vi "Sonatina.vi"(11 "NXT/EV3":T1) -> (3 "NXT/EV3 2":T1)   [LabVIEW 2016]
uses:
  <vilib>/NXT/Subs/LVHSConnector.ctl
  <vilib>/NXT/LegoClasses/BrickReference/BrickReference.lvclass
  <vilib>/NXT/Dual Mode Library/Display/drawText_Center.vi
  <vilib>/NXT/Dual Mode Library/Sound/PlayG.vi
  <vilib>/NXT/Dual Mode Library/Waits/Wait_Num.vi
  <vilib>/NXT/Dual Mode Library/Sound/PlayB.vi
  <vilib>/NXT/Dual Mode Library/Sound/PlayA.vi
  <vilib>/NXT/Dual Mode Library/Sound/PlayD.vi
  <vilib>/NXT/Dual Mode Library/Sound/PlayC.vi
  <vilib>/NXT/Dual Mode Library/Sound/PlayE.vi
  <vilib>/NXT/Dual Mode Library/Sound/PlayFsharp.vi
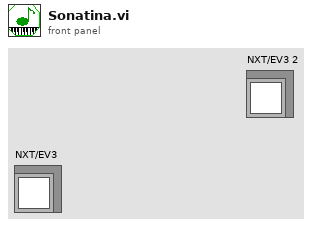
[diagram p1: front panel]
types:
  T1 = typedef "LVHSConnector.ctl" = refnum<class "BrickReference.lvclass">
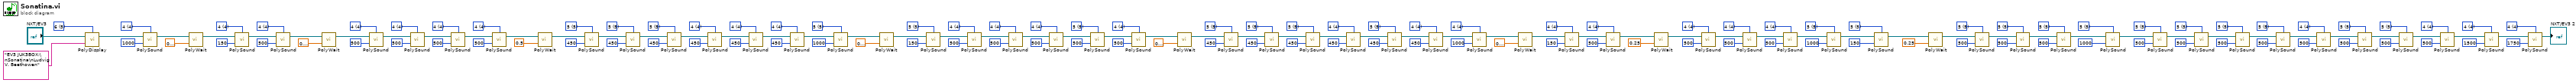
[diagram p0: block diagram]
diagram:
  w5 = u16 4 items=["3"=3, "4"=4, "5"=5, "6"=6, "7"=7] ("Octave")
  w9 = u16 5 items=["3"=3, "4"=4, "5"=5, "6"=6, "7"=7] ("Octave")
  w16 = u16 4 items=["3"=3, "4"=4, "5"=5, "6"=6, "7"=7] ("Octave")
  w19 = u16 4 items=["3"=3, "4"=4, "5"=5, "6"=6, "7"=7] ("Octave")
  w20 = u16 5 items=["3"=3, "4"=4, "5"=5, "6"=6, "7"=7] ("Octave")
  w23 = u16 4 items=["3"=3, "4"=4, "5"=5, "6"=6, "7"=7] ("Octave")
  w24 = u16 5 items=["3"=3, "4"=4, "5"=5, "6"=6, "7"=7] ("Octave")
  w27 = u16 5 items=["3"=3, "4"=4, "5"=5, "6"=6, "7"=7] ("Octave")
  w28 = u16 5 items=["3"=3, "4"=4, "5"=5, "6"=6, "7"=7] ("Octave")
  w31 = u16 5 items=["3"=3, "4"=4, "5"=5, "6"=6, "7"=7] ("Octave")
  w41 = u16 5 items=["3"=3, "4"=4, "5"=5, "6"=6, "7"=7] ("Octave")
  w40 = u16 5 items=["3"=3, "4"=4, "5"=5, "6"=6, "7"=7] ("Octave")
  w37 = u16 5 items=["3"=3, "4"=4, "5"=5, "6"=6, "7"=7] ("Octave")
  w36 = u16 5 items=["3"=3, "4"=4, "5"=5, "6"=6, "7"=7] ("Octave")
  w33 = u16 5 items=["3"=3, "4"=4, "5"=5, "6"=6, "7"=7] ("Octave")
  w61 = u16 5 items=["3"=3, "4"=4, "5"=5, "6"=6, "7"=7] ("Octave")
  w62 = u16 4 items=["3"=3, "4"=4, "5"=5, "6"=6, "7"=7] ("Octave")
  w65 = u16 4 items=["3"=3, "4"=4, "5"=5, "6"=6, "7"=7] ("Octave")
  w66 = u16 4 items=["3"=3, "4"=4, "5"=5, "6"=6, "7"=7] ("Octave")
  w69 = u16 4 items=["3"=3, "4"=4, "5"=5, "6"=6, "7"=7] ("Octave")
  w70 = u16 4 items=["3"=3, "4"=4, "5"=5, "6"=6, "7"=7] ("Octave")
  w73 = u16 4 items=["3"=3, "4"=4, "5"=5, "6"=6, "7"=7] ("Octave")
  w83 = u16 4 items=["3"=3, "4"=4, "5"=5, "6"=6, "7"=7] ("Octave")
  w84 = u16 5 items=["3"=3, "4"=4, "5"=5, "6"=6, "7"=7] ("Octave")
  w86 = u16 4 items=["3"=3, "4"=4, "5"=5, "6"=6, "7"=7] ("Octave")
  w89 = u16 5 items=["3"=3, "4"=4, "5"=5, "6"=6, "7"=7] ("Octave")
  w90 = u16 5 items=["3"=3, "4"=4, "5"=5, "6"=6, "7"=7] ("Octave")
  w93 = u16 5 items=["3"=3, "4"=4, "5"=5, "6"=6, "7"=7] ("Octave")
  w95 = u16 4 items=["3"=3, "4"=4, "5"=5, "6"=6, "7"=7] ("Octave")
  w110 = u16 5 items=["3"=3, "4"=4, "5"=5, "6"=6, "7"=7] ("Octave")
  w107 = u16 4 items=["3"=3, "4"=4, "5"=5, "6"=6, "7"=7] ("Octave")
  w106 = u16 4 items=["3"=3, "4"=4, "5"=5, "6"=6, "7"=7] ("Octave")
  w103 = u16 4 items=["3"=3, "4"=4, "5"=5, "6"=6, "7"=7] ("Octave")
  w102 = u16 5 items=["3"=3, "4"=4, "5"=5, "6"=6, "7"=7] ("Octave")
  w99 = u16 5 items=["3"=3, "4"=4, "5"=5, "6"=6, "7"=7] ("Octave")
  w123 = u16 4 items=["3"=3, "4"=4, "5"=5, "6"=6, "7"=7] ("Octave")
  w126 = u16 4 items=["3"=3, "4"=4, "5"=5, "6"=6, "7"=7] ("Octave")
  w130 = u16 4 items=["3"=3, "4"=4, "5"=5, "6"=6, "7"=7] ("Octave")
  w127 = u16 5 items=["3"=3, "4"=4, "5"=5, "6"=6, "7"=7] ("Octave")
  w133 = u16 5 items=["3"=3, "4"=4, "5"=5, "6"=6, "7"=7] ("Octave")
  w136 = u16 5 items=["3"=3, "4"=4, "5"=5, "6"=6, "7"=7] ("Octave")
  w149 = u16 4 items=["3"=3, "4"=4, "5"=5, "6"=6, "7"=7] ("Octave")
  w150 = u16 4 items=["3"=3, "4"=4, "5"=5, "6"=6, "7"=7] ("Octave")
  w153 = u16 4 items=["3"=3, "4"=4, "5"=5, "6"=6, "7"=7] ("Octave")
  w154 = u16 4 items=["3"=3, "4"=4, "5"=5, "6"=6, "7"=7] ("Octave")
  w157 = u16 4 items=["3"=3, "4"=4, "5"=5, "6"=6, "7"=7] ("Octave")
  w158 = u16 4 items=["3"=3, "4"=4, "5"=5, "6"=6, "7"=7] ("Octave")
  w161 = u16 4 items=["3"=3, "4"=4, "5"=5, "6"=6, "7"=7] ("Octave")
  w163 = i16 5 items=["1", "2", "3", "4", "5", "6", "7", "8", "9", "10", "11", "12"] ("Line")
  n1 = call-poly <vilib>:"PolyDisplay.vi"("Text"="EV3 JUK3BOX:\nSonatina\nLudvig V. Beethowen", "NXT/EV3"="NXT/EV3", "Line"=w163) -> ("NXT/EV3"=w143:T1)  [unwired: 1 in]
  n2 = call-poly <vilib>:"PolySound.vi"("Duration (500 ms)"=u16 1000, "NXT/EV3"=w143, "Octave"=w161) -> ("NXT/EV3"=w140:T1)  [unwired: 1 in]
  n3 = call-poly <vilib>:"PolyWait.vi"("Time (1 sec)"=sgl 0.1, "NXT/EV3"=w140) -> ("NXT/EV3"=w141:T1)  [unwired: 2 in]
  n4 = call-poly <vilib>:"PolySound.vi"("Duration (500 ms)"=u16 150, "NXT/EV3"=w141, "Octave"=w158) -> ("NXT/EV3"=w147:T1)  [unwired: 1 in]
  n5 = call-poly <vilib>:"PolySound.vi"("Duration (500 ms)"=u16 500, "NXT/EV3"=w147, "Octave"=w157) -> ("NXT/EV3"=w138:T1)  [unwired: 1 in]
  n6 = call-poly <vilib>:"PolyWait.vi"("Time (1 sec)"=sgl 0.1, "NXT/EV3"=w138) -> ("NXT/EV3"=w137:T1)  [unwired: 2 in]
  n7 = call-poly <vilib>:"PolySound.vi"("Duration (500 ms)"=u16 500, "NXT/EV3"=w137, "Octave"=w154) -> ("NXT/EV3"=w146:T1)  [unwired: 1 in]
  n8 = call-poly <vilib>:"PolySound.vi"("Duration (500 ms)"=u16 500, "NXT/EV3"=w146, "Octave"=w153) -> ("NXT/EV3"=w145:T1)  [unwired: 1 in]
  n9 = call-poly <vilib>:"PolySound.vi"("Duration (500 ms)"=u16 500, "NXT/EV3"=w145, "Octave"=w150) -> ("NXT/EV3"=w144:T1)  [unwired: 1 in]
  n10 = call-poly <vilib>:"PolySound.vi"("Duration (500 ms)"=u16 500, "NXT/EV3"=w144, "Octave"=w149) -> ("NXT/EV3"=w118:T1)  [unwired: 1 in]
  n11 = call-poly <vilib>:"PolyWait.vi"("Time (1 sec)"=sgl 0.5, "NXT/EV3"=w118) -> ("NXT/EV3"=w119:T1)  [unwired: 2 in]
  n12 = call-poly <vilib>:"PolySound.vi"("Duration (500 ms)"=u16 450, "NXT/EV3"=w119, "Octave"=w136) -> ("NXT/EV3"=w132:T1)  [unwired: 1 in]
  n13 = call-poly <vilib>:"PolySound.vi"("Duration (500 ms)"=u16 450, "NXT/EV3"=w132, "Octave"=w133) -> ("NXT/EV3"=w121:T1)  [unwired: 1 in]
  n14 = call-poly <vilib>:"PolySound.vi"("Duration (500 ms)"=u16 450, "NXT/EV3"=w121, "Octave"=w127) -> ("NXT/EV3"=w131:T1)  [unwired: 1 in]
  n15 = call-poly <vilib>:"PolySound.vi"("Duration (500 ms)"=u16 450, "NXT/EV3"=w131, "Octave"=w130) -> ("NXT/EV3"=w120:T1)  [unwired: 1 in]
  n16 = call-poly <vilib>:"PolySound.vi"("Duration (500 ms)"=u16 450, "NXT/EV3"=w120, "Octave"=w126) -> ("NXT/EV3"=w122:T1)  [unwired: 1 in]
  n17 = call-poly <vilib>:"PolySound.vi"("Duration (500 ms)"=u16 450, "NXT/EV3"=w122, "Octave"=w123) -> ("NXT/EV3"=w98:T1)  [unwired: 1 in]
  n18 = call-poly <vilib>:"PolySound.vi"("Duration (500 ms)"=u16 1000, "NXT/EV3"=w98, "Octave"=w99) -> ("NXT/EV3"=w116:T1)  [unwired: 1 in]
  n19 = call-poly <vilib>:"PolyWait.vi"("Time (1 sec)"=sgl 0.1, "NXT/EV3"=w116) -> ("NXT/EV3"=w115:T1)  [unwired: 2 in]
  n20 = call-poly <vilib>:"PolySound.vi"("Duration (500 ms)"=u16 150, "NXT/EV3"=w115, "Octave"=w102) -> ("NXT/EV3"=w111:T1)  [unwired: 1 in]
  n21 = call-poly <vilib>:"PolySound.vi"("Duration (500 ms)"=u16 500, "NXT/EV3"=w111, "Octave"=w103) -> ("NXT/EV3"=w97:T1)  [unwired: 1 in]
  n22 = call-poly <vilib>:"PolySound.vi"("Duration (500 ms)"=u16 500, "NXT/EV3"=w97, "Octave"=w106) -> ("NXT/EV3"=w112:T1)  [unwired: 1 in]
  n23 = call-poly <vilib>:"PolySound.vi"("Duration (500 ms)"=u16 500, "NXT/EV3"=w112, "Octave"=w107) -> ("NXT/EV3"=w113:T1)  [unwired: 1 in]
  n24 = call-poly <vilib>:"PolySound.vi"("Duration (500 ms)"=u16 500, "NXT/EV3"=w113, "Octave"=w110) -> ("NXT/EV3"=w94:T1)  [unwired: 1 in]
  n25 = call-poly <vilib>:"PolySound.vi"("Duration (500 ms)"=u16 500, "NXT/EV3"=w94, "Octave"=w95) -> ("NXT/EV3"=w76:T1)  [unwired: 1 in]
  n26 = call-poly <vilib>:"PolyWait.vi"("Time (1 sec)"=sgl 0.1, "NXT/EV3"=w76) -> ("NXT/EV3"=w75:T1)  [unwired: 2 in]
  n27 = call-poly <vilib>:"PolySound.vi"("Duration (500 ms)"=u16 450, "NXT/EV3"=w75, "Octave"=w93) -> ("NXT/EV3"=w81:T1)  [unwired: 1 in]
  n28 = call-poly <vilib>:"PolySound.vi"("Duration (500 ms)"=u16 450, "NXT/EV3"=w81, "Octave"=w90) -> ("NXT/EV3"=w80:T1)  [unwired: 1 in]
  n29 = call-poly <vilib>:"PolySound.vi"("Duration (500 ms)"=u16 450, "NXT/EV3"=w80, "Octave"=w89) -> ("NXT/EV3"=w79:T1)  [unwired: 1 in]
  n30 = call-poly <vilib>:"PolySound.vi"("Duration (500 ms)"=u16 450, "NXT/EV3"=w79, "Octave"=w86) -> ("NXT/EV3"=w74:T1)  [unwired: 1 in]
  n31 = call-poly <vilib>:"PolySound.vi"("Duration (500 ms)"=u16 450, "NXT/EV3"=w74, "Octave"=w84) -> ("NXT/EV3"=w78:T1)  [unwired: 1 in]
  n32 = call-poly <vilib>:"PolySound.vi"("Duration (500 ms)"=u16 450, "NXT/EV3"=w78, "Octave"=w83) -> ("NXT/EV3"=w50:T1)  [unwired: 1 in]
  n33 = call-poly <vilib>:"PolySound.vi"("Duration (500 ms)"=u16 1000, "NXT/EV3"=w50, "Octave"=w73) -> ("NXT/EV3"=w54:T1)  [unwired: 1 in]
  n34 = call-poly <vilib>:"PolyWait.vi"("Time (1 sec)"=sgl 0.1, "NXT/EV3"=w54) -> ("NXT/EV3"=w55:T1)  [unwired: 2 in]
  n35 = call-poly <vilib>:"PolySound.vi"("Duration (500 ms)"=u16 150, "NXT/EV3"=w55, "Octave"=w70) -> ("NXT/EV3"=w59:T1)  [unwired: 1 in]
  n36 = call-poly <vilib>:"PolySound.vi"("Duration (500 ms)"=u16 500, "NXT/EV3"=w59, "Octave"=w69) -> ("NXT/EV3"=w52:T1)  [unwired: 1 in]
  n37 = call-poly <vilib>:"PolyWait.vi"("Time (1 sec)"=sgl 0.25, "NXT/EV3"=w52) -> ("NXT/EV3"=w51:T1)  [unwired: 2 in]
  n38 = call-poly <vilib>:"PolySound.vi"("Duration (500 ms)"=u16 500, "NXT/EV3"=w51, "Octave"=w66) -> ("NXT/EV3"=w58:T1)  [unwired: 1 in]
  n39 = call-poly <vilib>:"PolySound.vi"("Duration (500 ms)"=u16 500, "NXT/EV3"=w58, "Octave"=w65) -> ("NXT/EV3"=w57:T1)  [unwired: 1 in]
  n40 = call-poly <vilib>:"PolySound.vi"("Duration (500 ms)"=u16 500, "NXT/EV3"=w57, "Octave"=w62) -> ("NXT/EV3"=w49:T1)  [unwired: 1 in]
  n41 = call-poly <vilib>:"PolySound.vi"("Duration (500 ms)"=u16 1000, "NXT/EV3"=w49, "Octave"=w61) -> ("NXT/EV3"=w32:T1)  [unwired: 1 in]
  n42 = call-poly <vilib>:"PolySound.vi"("Duration (500 ms)"=u16 150, "NXT/EV3"=w32, "Octave"=w33) -> ("NXT/EV3"=w46:T1)  [unwired: 1 in]
  n43 = call-poly <vilib>:"PolyWait.vi"("Time (1 sec)"=sgl 0.25, "NXT/EV3"=w46) -> ("NXT/EV3"=w47:T1)  [unwired: 2 in]
  n44 = call-poly <vilib>:"PolySound.vi"("Duration (500 ms)"=u16 500, "NXT/EV3"=w47, "Octave"=w36) -> ("NXT/EV3"=w43:T1)  [unwired: 1 in]
  n45 = call-poly <vilib>:"PolySound.vi"("Duration (500 ms)"=u16 500, "NXT/EV3"=w43, "Octave"=w37) -> ("NXT/EV3"=w44:T1)  [unwired: 1 in]
  n46 = call-poly <vilib>:"PolySound.vi"("Duration (500 ms)"=u16 500, "NXT/EV3"=w44, "Octave"=w40) -> ("NXT/EV3"=w48:T1)  [unwired: 1 in]
  n47 = call-poly <vilib>:"PolySound.vi"("Duration (500 ms)"=u16 1000, "NXT/EV3"=w48, "Octave"=w41) -> ("NXT/EV3"=w2:T1)  [unwired: 1 in]
  n48 = call-poly <vilib>:"PolySound.vi"("Duration (500 ms)"=u16 500, "NXT/EV3"=w2, "Octave"=w31) -> ("NXT/EV3"=w15:T1)  [unwired: 1 in]
  n49 = call-poly <vilib>:"PolySound.vi"("Duration (500 ms)"=u16 500, "NXT/EV3"=w15, "Octave"=w28) -> ("NXT/EV3"=w14:T1)  [unwired: 1 in]
  n50 = call-poly <vilib>:"PolySound.vi"("Duration (500 ms)"=u16 500, "NXT/EV3"=w14, "Octave"=w27) -> ("NXT/EV3"=w13:T1)  [unwired: 1 in]
  n51 = call-poly <vilib>:"PolySound.vi"("Duration (500 ms)"=u16 500, "NXT/EV3"=w13, "Octave"=w24) -> ("NXT/EV3"=w12:T1)  [unwired: 1 in]
  n52 = call-poly <vilib>:"PolySound.vi"("Duration (500 ms)"=u16 500, "NXT/EV3"=w12, "Octave"=w23) -> ("NXT/EV3"=w11:T1)  [unwired: 1 in]
  n53 = call-poly <vilib>:"PolySound.vi"("Duration (500 ms)"=u16 500, "NXT/EV3"=w11, "Octave"=w20) -> ("NXT/EV3"=w7:T1)  [unwired: 1 in]
  n54 = call-poly <vilib>:"PolySound.vi"("Duration (500 ms)"=u16 500, "NXT/EV3"=w7, "Octave"=w9) -> ("NXT/EV3"=w6:T1)  [unwired: 1 in]
  n55 = call-poly <vilib>:"PolySound.vi"("Duration (500 ms)"=u16 500, "NXT/EV3"=w6, "Octave"=w19) -> ("NXT/EV3"=w10:T1)  [unwired: 1 in]
  n56 = call-poly <vilib>:"PolySound.vi"("Duration (500 ms)"=u16 1500, "NXT/EV3"=w10, "Octave"=w16) -> ("NXT/EV3"=w3:T1)  [unwired: 1 in]
  n57 = call-poly <vilib>:"PolySound.vi"("Duration (500 ms)"=u16 1750, "NXT/EV3"=w3, "Octave"=w5) -> ("NXT/EV3"=→"NXT/EV3 2":T1)  [unwired: 1 in]
